vi "Server_main.vi"() -> ()   [LabVIEW 2020]
panel:
  out "Check data in SQL":string[][](array[string])
  in  "Export data":bool
  out "Data of user":string[][](array[string])
  in  "Port 1":u16
  in  "Port 2":u16
  in  "End Server":bool
  out "DATA":string
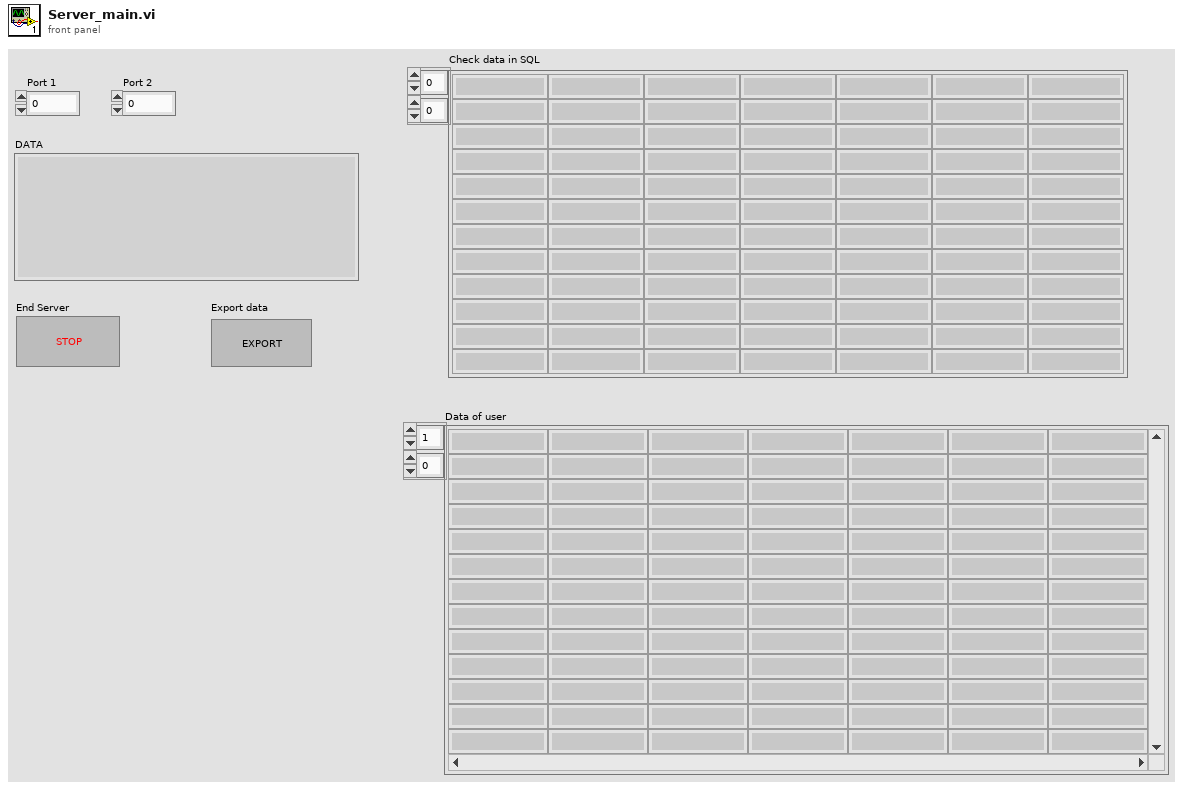
[diagram p1: front panel]
types:
  T1 = enum16{"Standard", "Buffered", "CRLF", "Immediate"}
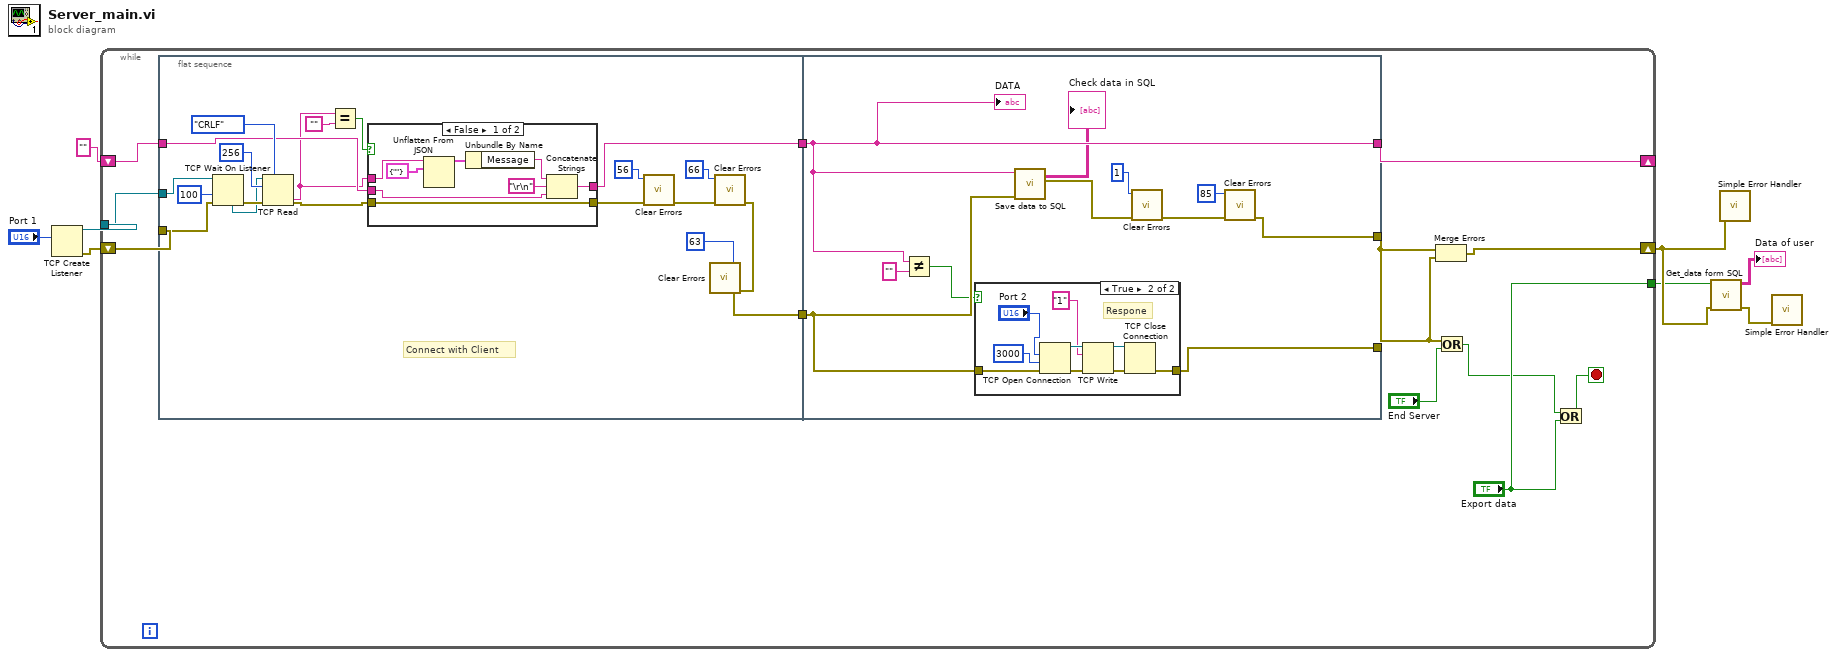
[diagram p0: block diagram]
diagram:
  n1 = TCP Create Listener(10:"Port 1") -> (0:w8:errorcluster, 3:w7:refnum<k5>)  [unwired: 4 in, 1 out]
  n2 = while {
    tunnel: w7 -> [w19]
    shift-right: [w13] -> w3
    shift-left: w8 -> [w20]
    shift-right: [w17] -> _
    shift-left: "" -> [w18]
    tunnel: ["Export data"] -> w1
    stop <- w9 stop-if-true
    n3 = flat-sequence {
      tunnel: w20 -> [w40]
      tunnel: w19 -> [w39]
      tunnel: w18 -> [w34]
      tunnel: [w33] -> w15
      tunnel: [w23] -> w14
      tunnel: [w54] -> w12
      tunnel: [w57] -> w17
      tunnel: w15 -> [w57]
      tunnel: w14 -> [w59]
      tunnel: [w60] -> _
      frame #0 {
        # "Connect with Client"
        n4 = TCP Wait On Listener(8:w40, 9:100 ("timeout ms (wait forever: -1)"), 11:w39) -> (0:w37:errorcluster, 4:w25:refnum<k5>)  [unwired: 1 in, 3 out]
        n5 = TCP Read(connection ID=w25, bytes to read=256, error in (no error)=w37, 7:T1."CRLF" ("mode (standard)")) -> (data out=w27:string, error out=w35:errorcluster)  [unwired: 1 in, 1 out]
        n6 = Equal?(x=w27, y="") -> (x = y?=w28:bool)
        n7 = case shown="False" w28 {
          tunnel: [w46 w50] -> w33
          tunnel: w27 -> [w45 _]
          tunnel: w35 -> [w41 w49]
          tunnel: w34 -> [w48 w50]
          tunnel: [w41 w49] -> w31
          frame False {
            n8 = Unflatten From JSON(JSON string=w45, type and defaults=cluster{"Message":string} {"Message"=""}) -> (value=w43:cluster{"Message":string})  [unwired: 5 in, 1 out]
            n9 = Unbundle By Name(w43) -> ("Message"=w42:string)
            n10 = Concatenate Strings(w42, "\r\n", w48) -> (w46:string)
          }
          frame True {
          }
        }
        n11 = call <vilib>:"Clear Errors.vi"("error in (no error)"=w31, "specific error code to clear (0: all)"=56) -> ("error out"=w32:errorcluster)  [unwired: 4 in, 1 out]
        n12 = call <vilib>:"Clear Errors.vi"("error in (no error)"=w32, "specific error code to clear (0: all)"=66) -> ("error out"=w22:errorcluster)  [unwired: 4 in, 1 out]
        n13 = call <vilib>:"Clear Errors.vi"("error in (no error)"=w22, "specific error code to clear (0: all)"=63) -> ("error out"=w23:errorcluster)  [unwired: 4 in, 1 out]
      }
      frame #1 {
        n14 = Not Equal?(x=w57, y="") -> (x != y?=w58:bool)
        n15 = case shown="True" w58 {
          tunnel: [w62 w67] -> w60
          tunnel: w59 -> [w62 w66]
          frame False {
          }
          frame True {
            # "Respone"
            n16 = TCP Open Connection(remote port or service name="Port 2", timeout ms (60000)=3000, error in (no error)=w66) -> (connection ID=w71:refnum<k5>, error out=w68:errorcluster)  [unwired: 2 in]
            n17 = TCP Write(connection ID=w71, data in="1", error in (no error)=w68) -> (connection ID out=w70:refnum<k5>, error out=w69:errorcluster)  [unwired: 1 in, 1 out]
            n18 = TCP Close Connection(connection ID=w70, error in (no error)=w69) -> (error out=w67:errorcluster)  [unwired: 1 in, 1 out]
          }
        }
        n19 = call "Save data to SQL.vi"("error in (no error)"=w59, "data in"=w57) -> ("Error out sql"=w56:errorcluster, "Data"=→"Check data in SQL":string[][])  [unwired: 8 in]
        n20 = call <vilib>:"Clear Errors.vi"("error in (no error)"=w56, "specific error code to clear (0: all)"=1) -> ("error out"=w53:errorcluster)  [unwired: 4 in, 1 out]
        n21 = call <vilib>:"Clear Errors.vi"("error in (no error)"=w53, "specific error code to clear (0: all)"=85) -> ("error out"=w54:errorcluster)  [unwired: 4 in, 1 out]
        "DATA" <- w57
      }
    }
    n22 = Merge Errors(w12, w12) -> (w13:errorcluster)
    n23 = Or(x=w12, y="End Server") -> (x .or. y?=w10:bool)
    n24 = Or(x=w10, y="Export data") -> (x .or. y?=w9:bool)
  }
  n25 = call "Get_data form SQL.vi"("error in (no error)"=w3, "Export"=w1) -> ("error out"=w2:errorcluster, "data"=→"Data of user":string[][])  [unwired: 8 in]
  n26 = call <vilib>:"Simple Error Handler.vi"("error in (no error)"=w3) -> ()  [unwired: 4 in, 5 out]
  n27 = call <vilib>:"Simple Error Handler.vi"("error in (no error)"=w2) -> ()  [unwired: 4 in, 5 out]
